vi "Image Acquiring Module.vi"(6 "#B scans":u32=1300, 7 "Scan Status in":enum16{"Start", "Continue Scan", "Finish Scan"}(ring), 8 "Error in":errorcluster, 10 "Channel":u32(ring)=1 items=["A"=1, "B"=2, "A + B"=3, "C"=4, "A + C"=5, "A + B"=6, "D"=8, "A + D"=9, "B + D"=10, "C + D"=12, "A + B + C + D"=15]) -> (0 "Error Out":errorcluster)   [LabVIEW 2018]
uses:
  Controls/FGV Actions.ctl
  Controls/QueueNames.ctl
  Controls/MessagePacket.ctl
  Controls/Queue Manager Actions.ctl
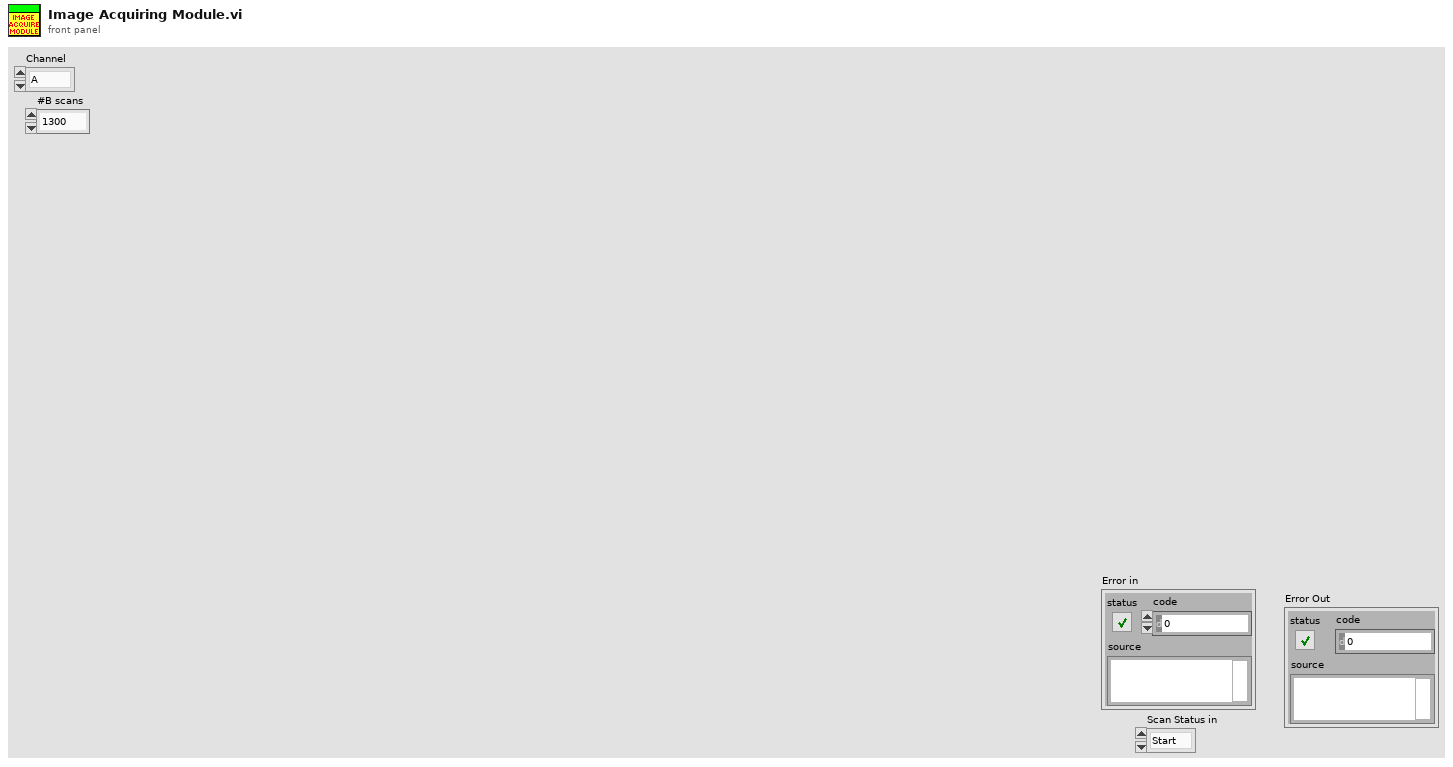
[diagram p1: front panel]
types:
  T1 = typedef "FGV Actions.ctl" = enum16{"Init", "Set", "Get", "Clear"}
  T2 = typedef "Queue Manager Actions.ctl" = enum16{"Init", "Enqueue", "Enqueue All", "Preview Queue", "Dequeue", "Get Status", "Flush Queue", "Flush All Queues", "Release All Queues", "Release Queue", "Enqueue at Opposite End"}
  T3 = typedef "MessagePacket.ctl" = cluster{"Message":string, "Parameter":variant}
  T4 = typedef "QueueNames.ctl" = enum16{"Main GUI", "Main Scan Processor", "Main Processing", "Main Saving", "Main Display", "Main Table Stage GUI", "Main Table Stage Proc.", "Scan Engine", "Vibratome GUI", "Vibratome Processor", "Slice Engine"}
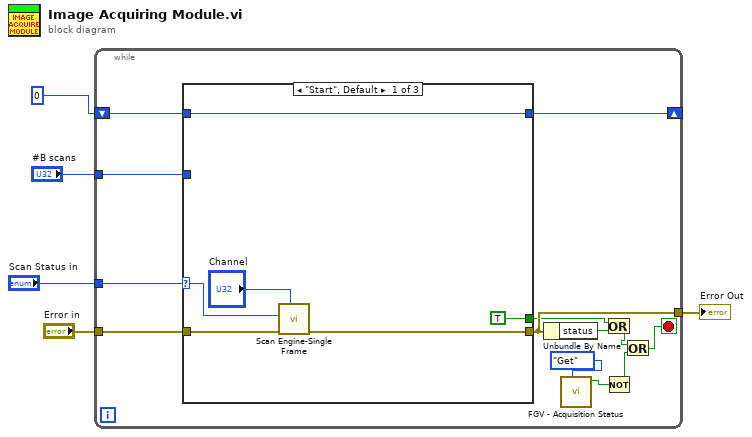
[diagram p0: block diagram]
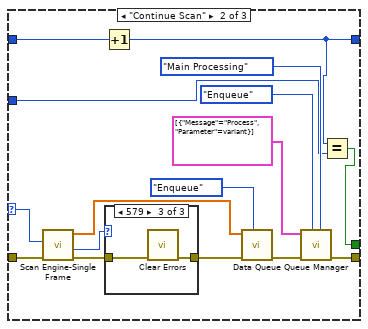
[diagram p2: hidden frame]
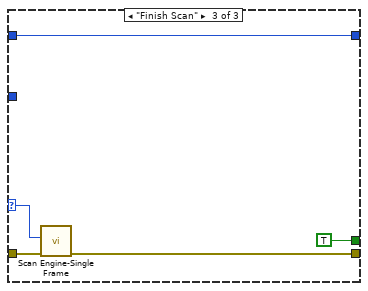
[diagram p5: hidden frame]
diagram:
  n1 = while {
    tunnel: "Error in" -> [w16]
    tunnel: "Scan Status in" -> [w18]
    tunnel: [w15] -> w3
    shift-right: [w17] -> _
    shift-left: u32 0 ("t") -> [w12]
    tunnel: "#B scans" -> [w6]
    stop <- w10 stop-if-true
    n2 = case shown="\"Start\", Default" w18 {
      selector: w18 -> [w23 w39 w49]
      tunnel: w16 -> [w24 w40 w48]
      tunnel: [w21 w38 w45] -> w15
      tunnel: [TRUE w26 TRUE ("task done?")] -> w13
      tunnel: w12 -> [w19 w32 w46]
      tunnel: [w19 w27 w46] -> w17
      tunnel: w6 -> [_ w25 _]
      frame "Start", Default {
        n3 = call "Scan Engine-Single Frame.vi"("Channel"="Channel", "Error in"=w24, "Scan Status"=w23) -> ("Error Out"=w21:errorcluster)  [unwired: 5 in, 3 out]
      }
      frame "Continue Scan" {
        n4 = call "Scan Engine-Single Frame.vi"("Error in"=w40, "Scan Status"=w39) -> ("Error Out"=w31:errorcluster, "Return Code"=w29:u32, "data out float"=w28:sgl[])  [unwired: 6 in, 1 out]
        n5 = Increment(x=w32) -> (x+1=w27:u32)
        n6 = case shown="579" w29 {
          tunnel: w31 -> [w41 w42 w44]
          tunnel: [w41 w42 w43] -> w30
          frame 0 {
          }
          frame 1, Default {
          }
          frame 579 {
            n7 = call <vilib>:"Clear Errors.vi"("error in (no error)"=w44) -> ("error out"=w43:errorcluster)  [unwired: 5 in, 1 out]
          }
        }
        n8 = call "Data Queue.vi"("Action"=Queue_Manager_Actions."Enqueue", "error in (no error)"=w30, "data in"=w28) -> ("error out"=w33:errorcluster)  [unwired: 6 in, 2 out]
        n9 = call "Queue Manager.vi"("Queue Name"=QueueNames."Main Processing", "Action"=Queue_Manager_Actions."Enqueue", "Error In"=w33, "Message Packet Array"=T3[] [{"Message"="Process", "Parameter"=variant}]) -> ("Error Out"=w38:errorcluster)  [unwired: 3 in, 4 out]
        n10 = Equal?(x=w27, y=w25) -> (x = y?=w26:bool)
      }
      frame "Finish Scan" {
        n11 = call "Scan Engine-Single Frame.vi"("Error in"=w48, "Scan Status"=w49) -> ("Error Out"=w45:errorcluster)  [unwired: 6 in, 3 out]
      }
    }
    n12 = Unbundle By Name(w15) -> ("status"=w14:bool)
    n13 = call "FGV - Acquisition Status.vi"("Actions"=FGV_Actions."Get") -> ("Level Status Out"=w8:bool)  [unwired: 6 in, 4 out]
    n14 = Or(x=w13, y=w14) -> (x .or. y?=w11:bool)
    n15 = Not(x=w8) -> (.not. x?=w7:bool)
    n16 = Or(x=w11, y=w7) -> (x .or. y?=w10:bool)
  }
  "Error Out" <- w3
